vi "nmea-line-from-buffer.vi"(5 "buffer":string) -> (0 "line":string, 1 "new line?":bool, 2 "remaining buffer":string)   [LabVIEW 2010]
uses:
  <vilib>/regexp/Match Regular Expression.xnode
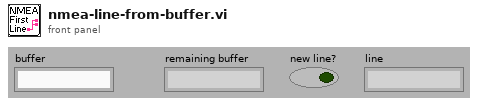
[diagram p1: front panel]
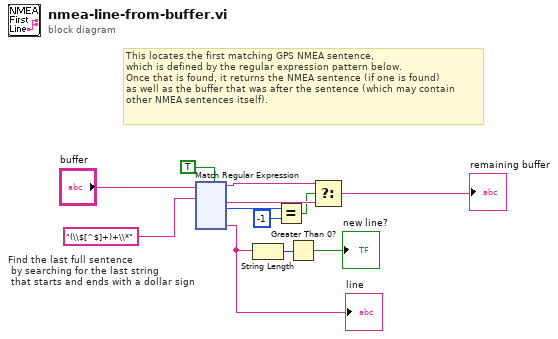
[diagram p0: block diagram]
diagram:
  w9 = "(\\$[^$]+)+\\*"  # Find the last full sentence  by searching for the last string  that starts and ends with a dollar sign
  # "This locates the first matching GPS NMEA sentence,\nwhich is defined by the regular expression pattern below.\nOnce that is found, it returns the NMEA sentence (if one is found)\nas well as the buffer that was after the sentence (which may contain\nother NMEA sentences itself)."
  n1 = xnode "Match Regular Expression"("input string"="buffer", "regular expression"=w9, "multiline? (F)"=TRUE) -> ("before match"=w5:string, "after match"=w4:string, "offset past match"=w6:i32, "submatch 1"=w2:string)  [unwired: 2 in, 3 out]
  "line" <- w2
  n2 = String Length(string=w2) -> (length=w7:i32)
  n3 = Equal?(x=w6, y=-1) -> (x = y?=w1:bool)
  n4 = Greater Than 0?(x=w7) -> (x > 0?=→"new line?":bool)
  n5 = Select(t=w5, s=w1, f=w4) -> (s? t:f=→"remaining buffer":string)
